vi "getElementText.vi"(8 "error in (no error)":errorcluster, 11 "Paragraph in":refnum<k24>) -> (0 "error out":errorcluster, 1 "Style":refnum<class "Style.lvclass">, 2 "Text":string, 3 "Paragraph out":refnum<k24>)   [LabVIEW 2017, in "xwpfReader.lvclass"]
uses:
  xwpfReader.lvclass
  C:/Users/Neo/Desktop/Dev_Tools_BR/LabVIEW_NPOI/src/lib/NPOI 2.1.1/NPOI.OOXML.dll
  lib/NPOI 2.1.1/NPOI.OOXML.dll
  Styles/Style/Style.lvclass
  Styles/Font--cluster.ctl
  Styles/Underline--ring.ctl
  Styles/Alignment--ring.ctl
  Styles/Styles.lvlib
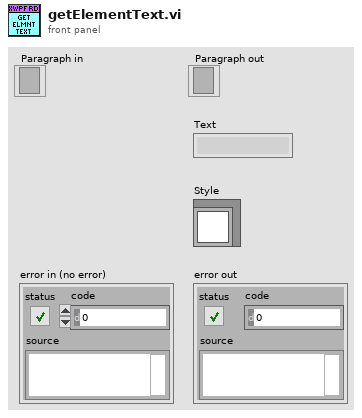
[diagram p1: front panel]
types:
  T1 = typedef "Styles.lvlib/Font--cluster.ctl" = cluster{"Name":string, "Size":i32, "Bold":bool, "Italic":bool, "Underline":T2, "Strike":bool, "Color":u32, "Alignment":T3}
  T2 = typedef "Styles.lvlib/Underline--ring.ctl" = i32
  T3 = typedef "Styles.lvlib/Alignment--ring.ctl" = i32
  T4 = cluster{"Text":string, "Style out":refnum<class "Style.lvclass">}
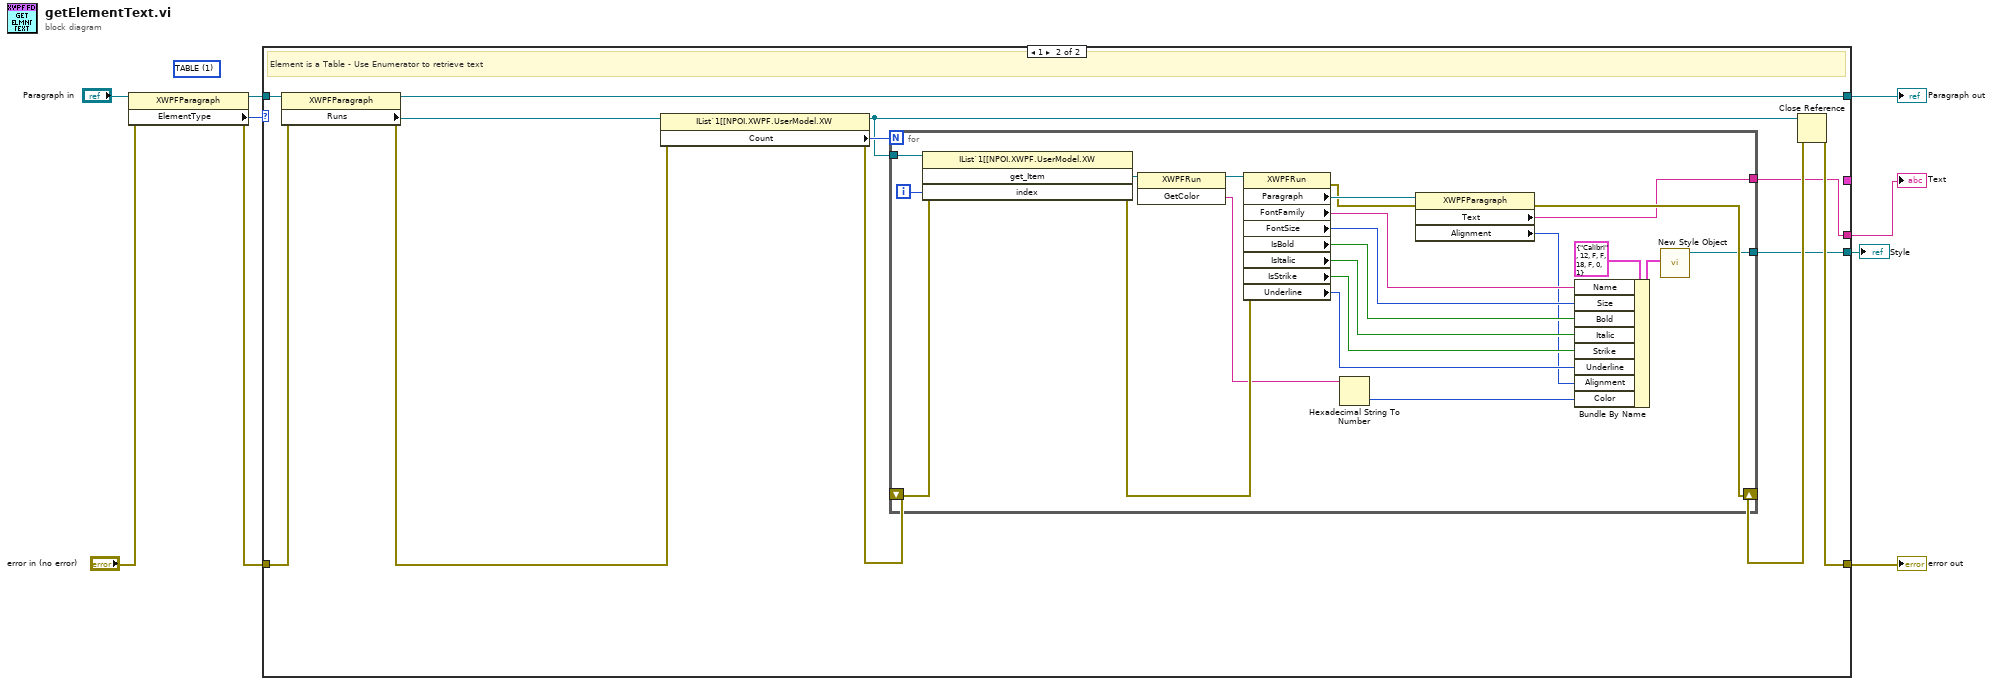
[diagram p0: block diagram]
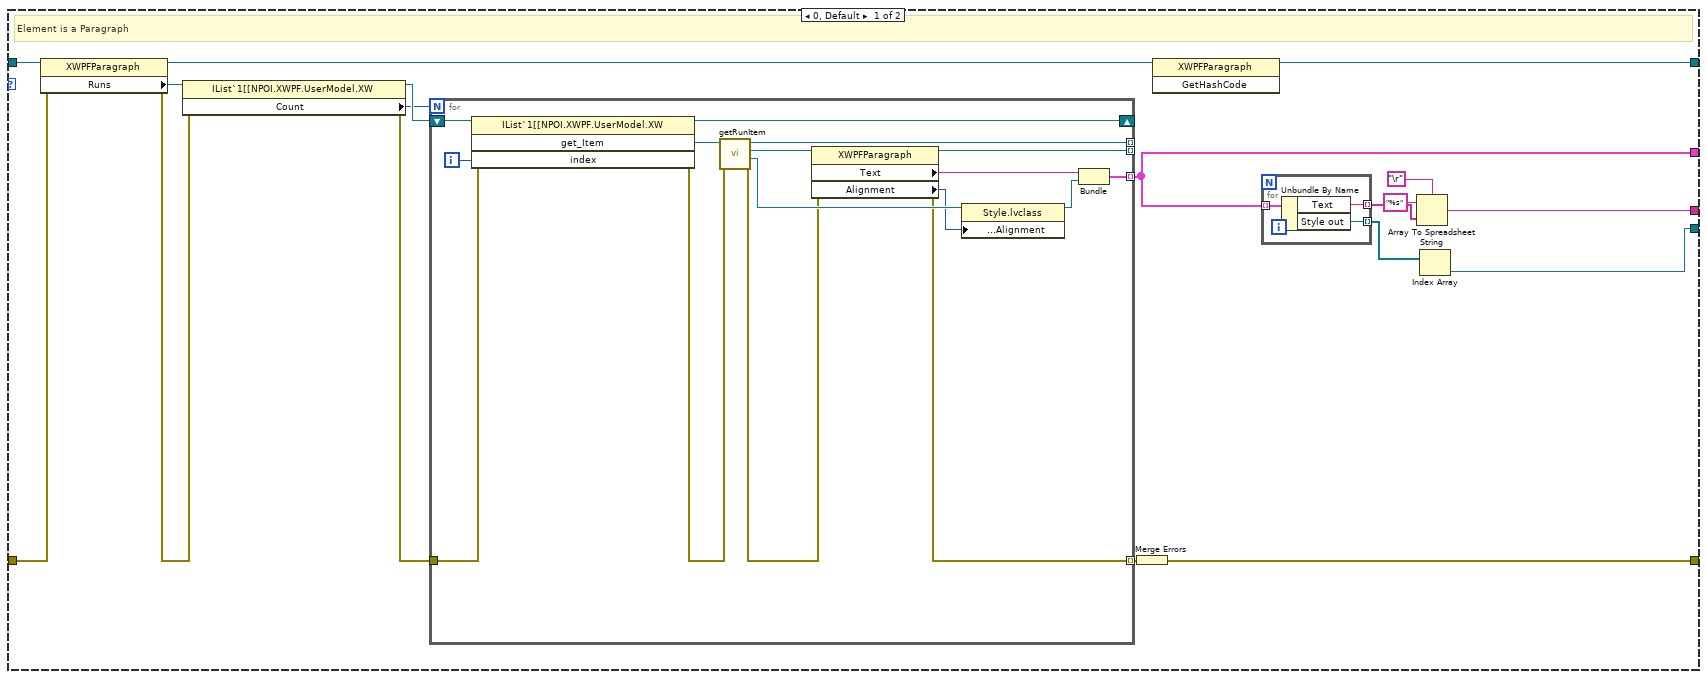
[diagram p2: hidden frame]
diagram:
  (unwired) 1 items=["PARAGRAPH", "TABLE"] ("ElementType")
  n1 = property class="XWPFParagraph"(reference="Paragraph in", error in="error in (no error)") -> (reference out=w7:refnum<k24>, error out=w5:errorcluster, "ElementType"=w8:i32)
  n2 = case shown="1" w8 {
    tunnel: w7 -> [w27 w58]
    tunnel: [w19 w57] -> w6
    tunnel: [w18 _] -> _
    tunnel: w5 -> [w23 w56]
    tunnel: [w10 w52] -> w4
    tunnel: [w12 w48] -> w3
    tunnel: [w14 w47] -> w1
    frame 0, Default {
      # "Element is a Paragraph"
      n3 = property class="XWPFParagraph"(reference=w27, error in=w23) -> (reference out=w20:refnum<k24>, error out=w22:errorcluster, "Runs"=w26:refnum<k24>)
      n4 = property class="IList`1[[NPOI.XWPF.UserModel.XW"(reference=w26, error in=w22) -> (reference out=w25:refnum<k24>, error out=w21:errorcluster, "Count"=w24:i32)
      n5 = for {
        N: w24 -> [_]
        tunnel: [w32] -> w18 mode=indexing
        tunnel: [w43] -> _ mode=indexing
        shift-right: [w40] -> _
        shift-left: w25 -> [w46]
        tunnel: w21 -> [w39]
        tunnel: [w35] -> w11 mode=indexing
        tunnel: [w31] -> _ mode=indexing
        i -> [w42]
        n6 = invoke class="IList`1[[NPOI.XWPF.UserModel.XW" method="get_Item"(reference=w46, error in=w39, "index"=w42) -> (reference out=w40:refnum<k24>, error out=w41:errorcluster, "get_Item"=w44:refnum<k24>)  [unwired: 1 in, 1 out]
        n7 = call "getRunItem.vi"("error in (no error)"=w41, "Run in"=w44) -> ("error out"=w36:errorcluster, "Style out"=w38:refnum<class "Style.lvclass">, "Paragraph"=w45:refnum<k24>, "Run out"=w43:refnum<k24>)  [unwired: 6 in]
        n8 = property class="XWPFParagraph"(reference=w45, error in=w36) -> (reference out=w31:refnum<k24>, error out=w35:errorcluster, "Text"=w34:string, "Alignment"=w37:i32)
        n9 = property class="Style.lvclass"(reference=w38, "Public VIs:Properties:Alignment"=w37) -> (reference out=w33:refnum<class "Style.lvclass">)  [unwired: 1 in, 1 out]
        n10 = Bundle("Text"=w34, "Style out"=w33) -> (w32:T4)  [unwired: 1 in]
      }
      n11 = Merge Errors(w11) -> (w10:errorcluster)
      n12 = invoke class="XWPFParagraph" method="GetHashCode"(reference=w20) -> (reference out=w19:refnum<k24>)  [unwired: 2 in, 2 out]
      n13 = for {
        tunnel: w18 -> [w30] mode=indexing
        tunnel: [w29] -> w17 mode=indexing
        tunnel: [w28] -> w13 mode=indexing
        n14 = Unbundle By Name(w30) -> ("Text"=w29:string, "Style out"=w28:refnum<class "Style.lvclass">)
      }
      n15 = Array To Spreadsheet String(delimiter (Tab)="\r", array=w17, 3:"%s" ("format string")) -> (spreadsheet string=w14:string)
      n16 = Index Array(array=w13) -> (element=w12:refnum<class "Style.lvclass">)  [unwired: 1 in]
    }
    frame 1 {
      # "Element is a Table - Use Enumerator to retrieve text"
      n17 = property class="XWPFParagraph"(reference=w58, error in=w56) -> (reference out=w57:refnum<k24>, error out=w55:errorcluster, "Runs"=w49:refnum<k24>)
      n18 = property class="IList`1[[NPOI.XWPF.UserModel.XW"(reference=w49, error in=w55) -> (reference out=w50:refnum<k24>, error out=w54:errorcluster, "Count"=w51:i32)
      n19 = for {
        N: w51 -> [_]
        tunnel: [w60] -> w47
        tunnel: w50 -> [w77]
        shift-right: [w62] -> w53
        shift-left: w54 -> [w78]
        tunnel: [w59] -> w48
        i -> [w76]
        n20 = invoke class="IList`1[[NPOI.XWPF.UserModel.XW" method="get_Item"(reference=w77, error in=w78, "index"=w76) -> (error out=w79:errorcluster, "get_Item"=w80:refnum<k24>)  [unwired: 1 in, 2 out]
        n21 = invoke class="XWPFRun" method="GetColor"(reference=w80) -> (reference out=w65:refnum<k24>, "GetColor"=w64:string)  [unwired: 2 in, 1 out]
        n22 = property class="XWPFRun"(reference=w65, error in=w79) -> (error out=w63:errorcluster, "Paragraph"=w75:refnum<k24>, "FontFamily"=w72:string, "FontSize"=w71:i32, "IsBold"=w70:bool, "IsItalic"=w69:bool, "IsStrike"=w68:bool, "Underline"=w67:i32)  [unwired: 1 out]
        n23 = Hexadecimal String To Number(string=w64) -> (number=w61:u32)  [unwired: 2 in, 1 out]
        n24 = property class="XWPFParagraph"(reference=w75, error in=w63) -> (error out=w62:errorcluster, "Text"=w60:string, "Alignment"=w66:i32)  [unwired: 1 out]
        n25 = Bundle By Name(cluster=T1 {"Name"="Calibri", "Size"=12, "Bold"=FALSE, "Italic"=FALSE, "Underline"=18, "Strike"=FALSE, "Color"=0, "Alignment"=1} ("Font"), "Name"=w72, "Size"=w71, "Bold"=w70, "Italic"=w69, "Strike"=w68, "Underline"=w67, "Alignment"=w66, "Color"=w61) -> (w73:T1)
        n26 = call "New Style Object.vi"("Font"=w73) -> ("Style out"=w59:refnum<class "Style.lvclass">)  [unwired: 9 in, 1 out]
      }
      n27 = Close Reference(reference=w50, error in (no error)=w53) -> (error out=w52:errorcluster)
    }
  }
  "error out" <- w4
  "Paragraph out" <- w6
  "Text" <- w1
  "Style" <- w3
